vi "Write Dev Grabber Config.vi"(8 "error in (no error)":errorcluster, 10 "Dev Grabber Config":T1, 11 "Dev Grabber in":refnum<class "Dev Grabber.lvclass">) -> (0 "error out":errorcluster, 3 "Dev Grabber out":refnum<class "Dev Grabber.lvclass">)   [LabVIEW 2014, in "Dev Grabber.lvlib" / "Dev Grabber.lvclass"]
uses:
  Dev Grabber.lvclass
  Dev Grabber Config.ctl
  <vilib>/Rock Robotics/WPI/Solenoid/WPI_SolenoidChannel.ctl
  Dev Grabber.lvclass/Dev Grabber.ctl
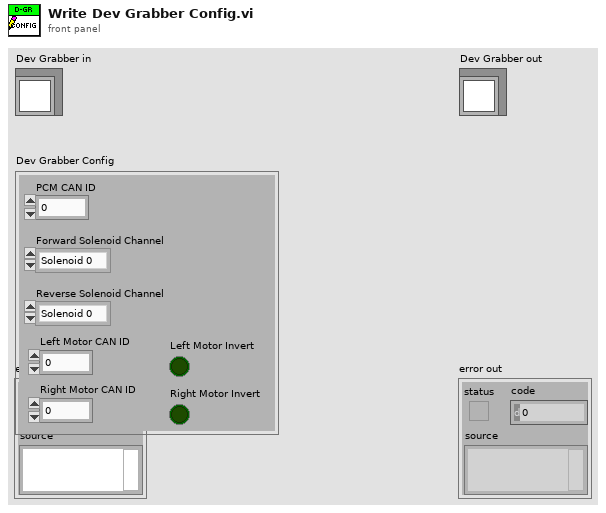
[diagram p1: front panel]
types:
  T1 = typedef "Dev Grabber.lvlib/Dev Grabber.lvclass/Dev Grabber Config.ctl" = cluster{"PCM CAN ID":u8, "Forward Solenoid Channel":T2, "Reverse Solenoid Channel":T2, "Left Motor CAN ID":u8, "Right Motor CAN ID":u8, "Left Motor Invert":bool, "Right Motor Invert":bool}
  T2 = typedef "WPI_SolenoidChannel.ctl" = enum8{"Solenoid 0", "Solenoid 1", "Solenoid 2", "Solenoid 3", "Solenoid 4", "Solenoid 5", "Solenoid 6", "Solenoid 7", "Invalid"}
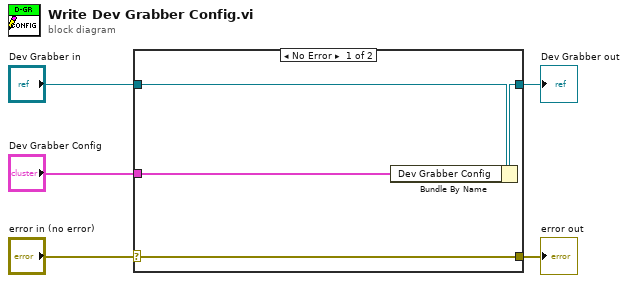
[diagram p0: block diagram]
diagram:
  n1 = case shown="No Error" "error in (no error)" {
    selector: "error in (no error)" -> [w9 w10]
    tunnel: [w9 w10] -> w4
    tunnel: [w7 w11] -> w2
    tunnel: "Dev Grabber in" -> [w8 w11]
    tunnel: "Dev Grabber Config" -> [w6 _]
    frame No Error {
      n2 = Bundle By Name(cluster=w8, "Dev Grabber Config"=w6) -> (w7:refnum<class "Dev Grabber.lvclass">)
    }
    frame Error {
    }
  }
  "error out" <- w4
  "Dev Grabber out" <- w2
